vi "hex string to decimal string.vi"(10 "Hex String":string) -> (2 "Decimal String":string)   [LabVIEW 8.6]
doc: "This VI convert hex string to decimal string."
panel:
  # "hex string to decimal string.vi\nConvert raw hex string to decimal string.\n\ncaozijian.cn@gmail.com"
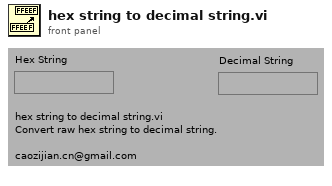
[diagram p1: front panel]
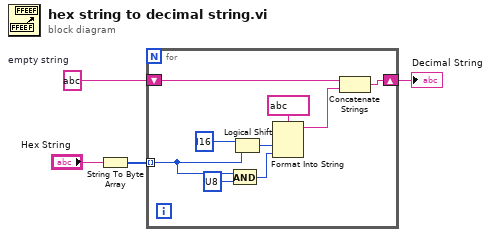
[diagram p0: block diagram]
diagram:
  w3 = string ?  # empty string
  n1 = String To Byte Array(string="Hex String") -> (unsigned byte array=w4:u8[])
  n2 = for {
    tunnel: w4 -> [w11] mode=indexing
    shift-right: [w5] -> w2
    shift-left: w3 -> [w7]
    n3 = And(x=w11, y=u8 ?) -> (x .and. y?=w8:u8)
    n4 = Logical Shift(y=i16 ?, x=w11) -> (x << y=w9:u8)
    n5 = Format Into String(format string=string ?, w9, w8) -> (resulting string=w6:string)  [unwired: 2 in, 1 out]
    n6 = Concatenate Strings(w7, w6) -> (w5:string)
  }
  "Decimal String" <- w2
